vi "Drive Core.vi"   [LabVIEW 2014]
uses:
  <vilib>/Rock Robotics/WPI/DriverStation/WPI_DriverStationRobotMode2.ctl
  Begin/Global Variables.vi
  Begin/Global Constants.vi
types:
  T1 = typedef "WPI_DriverStationRobotMode2.ctl" = enum16{"Autonomous Disabled", "Autonomous Enabled", "Teleop Disabled", "Teleop Enabled", "Disconnected", "Finish", "Test Disabled", "Test Enabled", "Emergency Stopped"}
  T2 = cluster{"Header P":dbl, "Header I":dbl, "Header D":dbl}
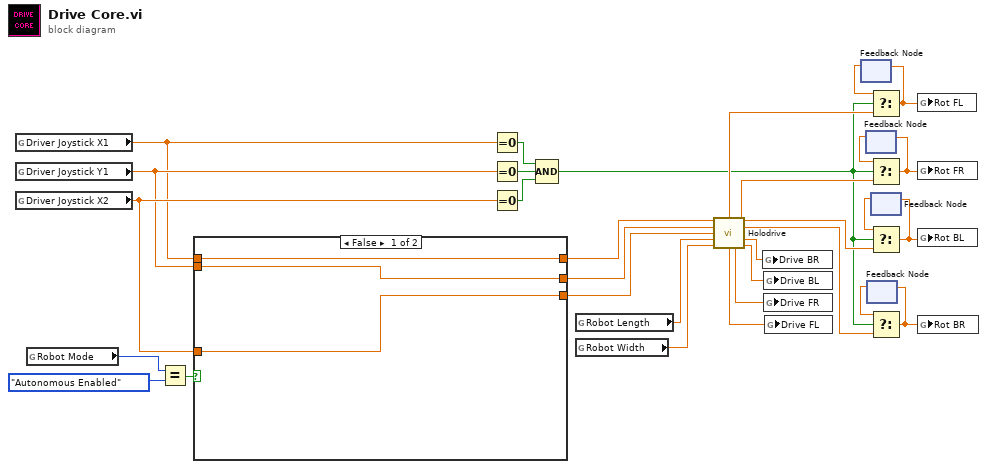
[diagram p0: block diagram]
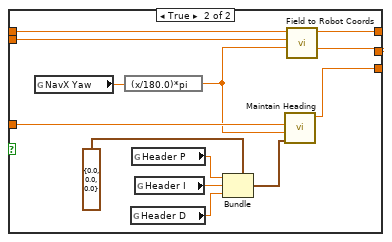
[diagram p2: hidden frame]
diagram:
  n1 = global read "Global Variables.vi" "Driver Joystick X1"() -> (w23:dbl)
  n2 = global read "Global Variables.vi" "Driver Joystick Y1"() -> (w24:dbl)
  n3 = global read "Global Variables.vi" "Driver Joystick X2"() -> (w28:dbl)
  n4 = global read "Global Variables.vi" "Robot Mode"() -> (w27:T1)
  n5 = Equal?(x=w27, y=WPI_DriverStationRobotMode2."Autonomous Enabled") -> (x = y?=w22:bool)
  n6 = case shown="False" w22 {
    tunnel: w23 -> [w34 w47]
    tunnel: w24 -> [w33 w46]
    tunnel: [w34 w45] -> w25
    tunnel: [w33 w44] -> w26
    tunnel: w28 -> [w32 w43]
    tunnel: [w32 w42] -> w29
    frame False {
    }
    frame True {
      n7 = global read "Global Variables.vi" "NavX Yaw"() -> (w41:dbl)
      n8 = expression code="(x/180.0)*pi" ("degrees to radians")(w41) -> (w40:dbl)
      n9 = global read "Global Constants.vi" "Header D"() -> (w37:dbl)
      n10 = global read "Global Constants.vi" "Header P"() -> (w39:dbl)
      n11 = global read "Global Constants.vi" "Header I"() -> (w38:dbl)
      n12 = Bundle(cluster=T2 {"Header P"=0.0, "Header I"=0.0, "Header D"=0.0}, "Header P"=w39, "Header I"=w38, "Header D"=w37) -> (w36:T2)
      n13 = call "Maintain Heading.vi"("PID gains"=w36, "NavX Yaw"=w40, "Raw Driver Joystick X2"=w43) -> ("Driver Joystick X2"=w42:dbl)  [unwired: 8 in]
      n14 = call "Field to Robot Coords.vi"("gyro"=w40, "Joystick y"=w46, "Joystick x"=w47) -> ("robot y"=w44:dbl, "robot x"=w45:dbl)  [unwired: 7 in]
    }
  }
  n15 = Equal To 0?(x=w23) -> (x = 0?=w5:bool)
  n16 = Equal To 0?(x=w24) -> (x = 0?=w6:bool)
  n17 = Equal To 0?(x=w28) -> (x = 0?=w7:bool)
  n18 = Compound Arithmetic op=AND(w5, w6, w7) -> (w8:bool)
  n19 = global read "Global Constants.vi" "Robot Length"() -> (w30:dbl)
  n20 = global read "Global Constants.vi" "Robot Width"() -> (w31:dbl)
  n21 = call "Holodrive.vi"("Translation X"=w25, "Translation Y"=w26, "Angular"=w29, "Robot Length"=w30, "Robot Width"=w31) -> ("FL Rot"=w14:dbl, "FR Rot"=w11:dbl, "BL Rot"=w12:dbl, "BR Rot"=w13:dbl, "BR Drive"=w4:dbl, "FL Drive"=w1:dbl, "FR Drive"=w2:dbl, "BL Drive"=w3:dbl)  [unwired: 3 in]
  n22 = global write "Global Variables.vi" "Drive BR"(w4) -> ()
  n23 = global write "Global Variables.vi" "Drive BL"(w3) -> ()
  n24 = global write "Global Variables.vi" "Drive FR"(w2) -> ()
  n25 = global write "Global Variables.vi" "Drive FL"(w1) -> ()
  n26 = feedback #1() -> (w16:dbl)  [unwired: 1 in]
  n27 = feedback #2() -> (w10:dbl)  [unwired: 1 in]
  n28 = feedback #3() -> (w20:dbl)  [unwired: 1 in]
  n29 = Select(t=w16, s=w8, f=w14) -> (s? t:f=w15:dbl)
  n30 = feedback-in #1(w15) -> ()
  n31 = Select(t=w10, s=w8, f=w11) -> (s? t:f=w9:dbl)
  n32 = feedback-in #2(w9) -> ()
  n33 = feedback #4() -> (w18:dbl)  [unwired: 1 in]
  n34 = Select(t=w18, s=w8, f=w12) -> (s? t:f=w17:dbl)
  n35 = feedback-in #4(w17) -> ()
  n36 = Select(t=w20, s=w8, f=w13) -> (s? t:f=w19:dbl)
  n37 = feedback-in #3(w19) -> ()
  n38 = global write "Global Variables.vi" "Rot FL"(w15) -> ()
  n39 = global write "Global Variables.vi" "Rot FR"(w9) -> ()
  n40 = global write "Global Variables.vi" "Rot BL"(w17) -> ()
  n41 = global write "Global Variables.vi" "Rot BR"(w19) -> ()
